vi "Error Handler.vi"(8 "error in (no error)":errorcluster, 9 "Status Code":u16, 10 "Status String":string, 11 "REST Client in":refnum<class "REST Client.lvclass">) -> (0 "error out":errorcluster, 3 "REST Client out":refnum<class "REST Client.lvclass">)   [LabVIEW 2013, in "REST Client.lvclass"]
uses:
  REST Client.lvclass
panel:
  # "Copyright © 2014 JKI All rights reserved.\n\nAuthor: Tomi Maila <tomi.maila@jki.net>\n\nThis library is provided \"AS IS\" ,WITHOUT WARRANTIES OR \nCONDITIONS OF ANY KIND, either express or implied.\n\nJKI -- jki.net"
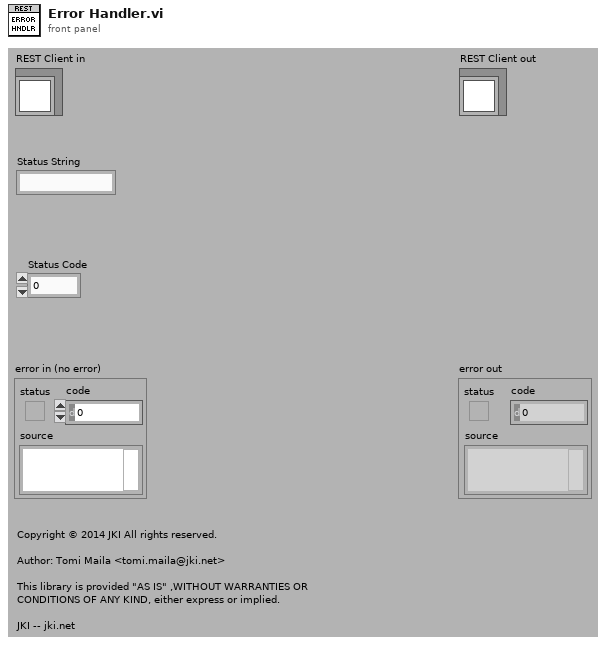
[diagram p1: front panel]
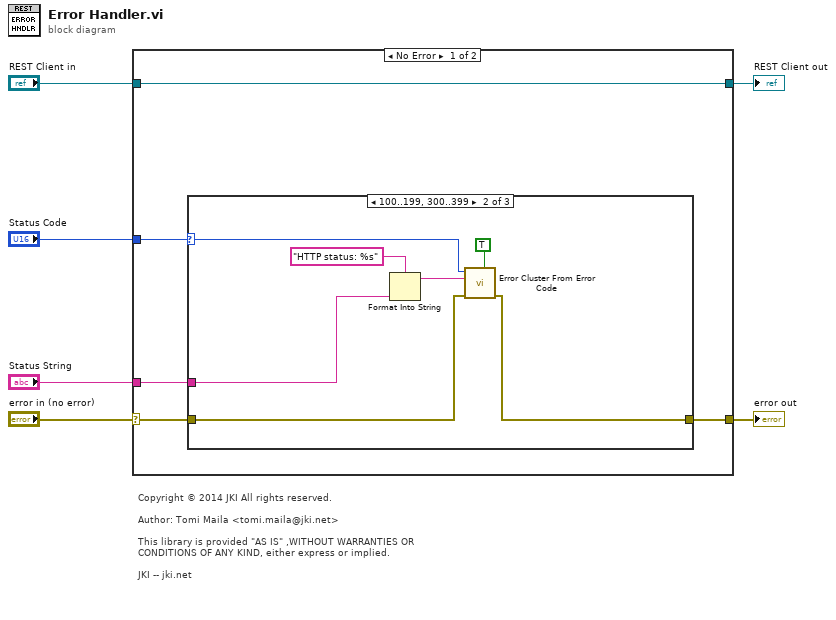
[diagram p0: block diagram]
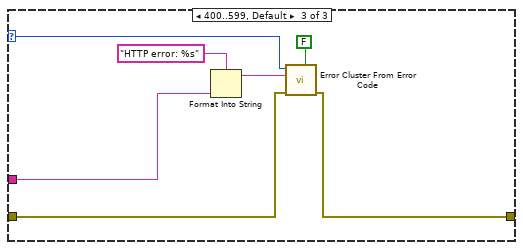
[diagram p3: hidden frame]
diagram:
  # "Copyright © 2014 JKI All rights reserved.\n\nAuthor: Tomi Maila <tomi.maila@jki.net>\n\nThis library is provided \"AS IS\" ,WITHOUT WARRANTIES OR \nCONDITIONS OF ANY KIND, either express or implied.\n\nJKI -- jki.net"
  n1 = case shown="No Error" "error in (no error)" {
    selector: "error in (no error)" -> [w8 w28]
    tunnel: [w7 w28] -> w5
    tunnel: [w11 w27] -> w3
    tunnel: "REST Client in" -> [w11 w27]
    tunnel: "Status Code" -> [w10 _]
    tunnel: "Status String" -> [w9 _]
    frame No Error {
      n2 = case shown="100..199, 300..399" w10 {
        selector: w10 -> [_ w17 w24]
        tunnel: w9 -> [_ w13 w20]
        tunnel: w8 -> [w12 w18 w25]
        tunnel: [w12 w19 w26] -> w7
        frame 200..299 {
          # "Expected response"
        }
        frame 100..199, 300..399 {
          n3 = Format Into String(format string="HTTP status: %s", w13) -> (resulting string=w14:string)  [unwired: 2 in, 1 out]
          n4 = call <vilib>:"Error Cluster From Error Code.vi"("is warning? (False)"=TRUE, "error in (no error)"=w18, "error message (\"\")"=w14, "error code (0)"=w17) -> ("error out"=w19:errorcluster)  [unwired: 5 in]
        }
        frame 400..599, Default {
          n5 = Format Into String(format string="HTTP error: %s", w20) -> (resulting string=w21:string)  [unwired: 2 in, 1 out]
          n6 = call <vilib>:"Error Cluster From Error Code.vi"("is warning? (False)"=FALSE, "error in (no error)"=w25, "error message (\"\")"=w21, "error code (0)"=w24) -> ("error out"=w26:errorcluster)  [unwired: 5 in]
        }
      }
    }
    frame Error {
    }
  }
  "error out" <- w5
  "REST Client out" <- w3
